vi "Clean CCD.vi"(8 "error in (no error)":errorcluster, 11 "CCD in":refnum<class "CCD.lvclass">) -> (0 "error out":errorcluster, 3 "CCD out":refnum<class "CCD.lvclass">)   [LabVIEW 2018, in "CCD.lvclass"]
uses:
  CCD.lvclass
  CCD.lvclass/CCD.ctl
panel:
  out "Cluster":T1
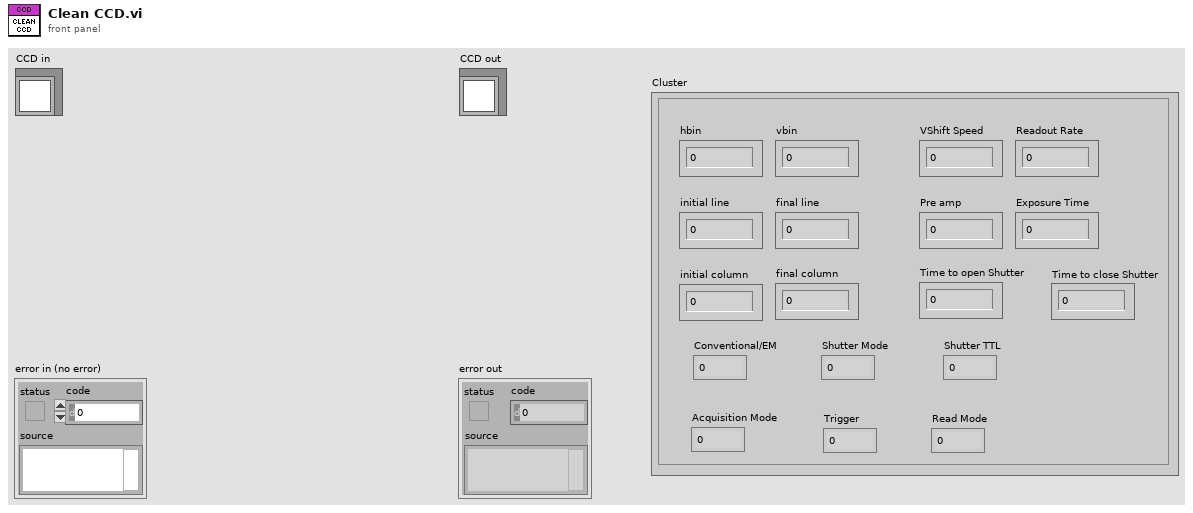
[diagram p1: front panel]
types:
  T1 = cluster{"hbin":u16, "vbin":u16, "initial line":u16, "final line":u16, "initial column":u16, "final column":u16, "VShift Speed":u8, "Readout Rate":u8, "Pre amp":u8, "Exposure Time":dbl, "Conventional/EM":u16, "Shutter Mode":u16, "Shutter TTL":u16, "Trigger":u16, "Time to open Shutter":u16, "Time to close Shutter":u16, "Acquisition Mode":u16, "Read Mode":u16}
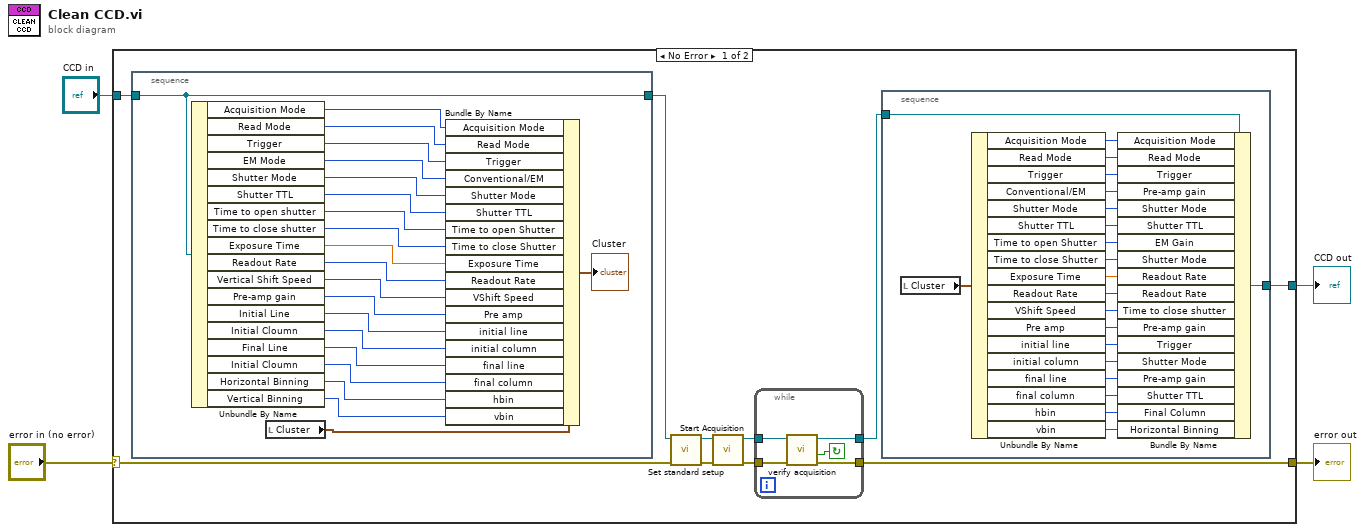
[diagram p0: block diagram]
diagram:
  n1 = case shown="No Error" "error in (no error)" {
    selector: "error in (no error)" -> [w11 w63]
    tunnel: "CCD in" -> [w14 w62]
    tunnel: [w5 w62] -> w2
    tunnel: [w6 w63] -> w1
    frame No Error {
      n2 = stacked-sequence {
        tunnel: w14 -> [w42]
        tunnel: [w42] -> w12
        frame #0 {
          n3 = Unbundle By Name(w42) -> ("Acquisition Mode"=w60:u8, "Read Mode"=w59:u8, "Trigger"=w58:u8, "EM Mode"=w57:u8, "Shutter Mode"=w56:u8, "Shutter TTL"=w55:u8, "Time to open shutter"=w54:u16, "Time to close shutter"=w53:u16, "Exposure Time"=w52:dbl, "Readout Rate"=w51:u8, "Vertical Shift Speed"=w50:u8, "Pre-amp gain"=w49:u8, "Initial Line"=w48:u16, "Initial Cloumn"=w47:u16, "Final Line"=w46:u16, "Initial Cloumn"=w45:u16, "Horizontal Binning"=w44:u16, "Vertical Binning"=w43:u16)
          n4 = local read "Cluster"() -> (w41:T1)
          n5 = Bundle By Name(cluster=w41, "Acquisition Mode"=w60, "Read Mode"=w59, "Trigger"=w58, "Conventional/EM"=w57, "Shutter Mode"=w56, "Shutter TTL"=w55, "Time to open Shutter"=w54, "Time to close Shutter"=w53, "Exposure Time"=w52, "Readout Rate"=w51, "VShift Speed"=w50, "Pre amp"=w49, "initial line"=w48, "initial column"=w47, "final line"=w46, "final column"=w45, "hbin"=w44, "vbin"=w43) -> (→"Cluster":T1)
        }
      }
      n6 = call "Set standard setup.vi"("error in (no error)"=w11, "CCD in"=w12) -> ("error out"=w9:errorcluster, "CCD out"=w10:refnum<class "CCD.lvclass">)  [unwired: 8 in]
      n7 = call "Start Acquisition.vi"("error in (no error)"=w9, "CCD in"=w10) -> ("error out"=w8:errorcluster, "CCD out"=w7:refnum<class "CCD.lvclass">)  [unwired: 8 in]
      n8 = while {
        tunnel: [w37] -> w6
        tunnel: [w38] -> w13
        tunnel: w8 -> [w39]
        tunnel: w7 -> [w40]
        stop <- w36 continue-if-true
        n9 = call "verify acquisition"("error in (no error)"=w39, "CCD in"=w40) -> ("error out"=w37:errorcluster, "Acquiring"=w36:bool, "CCD out"=w38:refnum<class "CCD.lvclass">)  [unwired: 7 in]
      }
      n10 = stacked-sequence {
        tunnel: w13 -> [w15]
        tunnel: [w17] -> w5
        frame #0 {
          n11 = local read "Cluster"() -> (w16:T1)
          n12 = Unbundle By Name(w16) -> ("Acquisition Mode"=w35:u16, "Read Mode"=w34:u16, "Trigger"=w33:u16, "Conventional/EM"=w32:u16, "Shutter Mode"=w31:u16, "Shutter TTL"=w30:u16, "Time to open Shutter"=w29:u16, "Time to close Shutter"=w28:u16, "Exposure Time"=w27:dbl, "Readout Rate"=w26:u8, "VShift Speed"=w25:u8, "Pre amp"=w24:u8, "initial line"=w23:u16, "initial column"=w22:u16, "final line"=w21:u16, "final column"=w20:u16, "hbin"=w19:u16, "vbin"=w18:u16)
          n13 = Bundle By Name(cluster=w15, "Acquisition Mode"=w35, "Read Mode"=w34, "Trigger"=w33, "Pre-amp gain"=w32, "Shutter Mode"=w31, "Shutter TTL"=w30, "EM Gain"=w29, "Shutter Mode"=w28, "Readout Rate"=w27, "Readout Rate"=w26, "Time to close shutter"=w25, "Pre-amp gain"=w24, "Trigger"=w23, "Shutter Mode"=w22, "Pre-amp gain"=w21, "Shutter TTL"=w20, "Final Column"=w19, "Horizontal Binning"=w18) -> (w17:refnum<class "CCD.lvclass">)
        }
      }
    }
    frame Error {
    }
  }
  "error out" <- w1
  "CCD out" <- w2
